vi "FTW-ERR-ThrowInvalidReferenceError.vi"(7 "Reference Type":string, 11 "error in":errorcluster) -> (15 "error out":errorcluster)   [LabVIEW 2014]
uses:
  FTW-ERR-NoErrorConstant.vi
  string/FTW-STR-ReplaceWhitespace.vi
  FTW-ERR-CallChain.vi
panel:
  # "Inputs"
  # "Outputs"
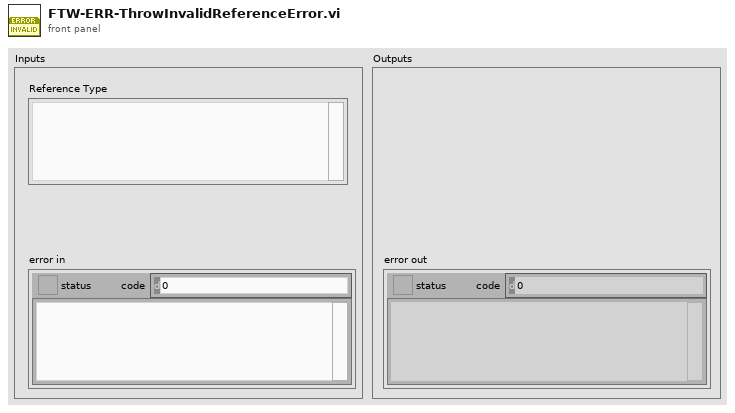
[diagram p1: front panel]
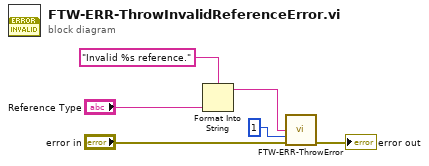
[diagram p0: block diagram]
diagram:
  n1 = Format Into String(format string="Invalid %s reference.", "Reference Type") -> (resulting string=w2:string)  [unwired: 2 in, 1 out]
  n2 = call "FTW-ERR-ThrowError.vi"("Error Message"=w2, "Error Code"=1 ("code"), "error in"="error in") -> ("error out"=→"error out":errorcluster)  [unwired: 12 in]
